vi "input.vi"(8 "error in":errorcluster, 10 "data table in":T1, 11 "Scan Engine runtime in":refnum<class "Scan Engine runtime.lvclass">) -> (0 "error out":errorcluster, 2 "data table out":T1, 3 "Scan Engine runtime out":refnum<class "Scan Engine runtime.lvclass">)   [LabVIEW 2014, in "Scan Engine runtime.lvclass"]
doc: "Provides an interface for reading data from a module at runtime. While this interface performs no operations, a child should provide an override which may read from any open sessions, references, or interfaces."
uses:
  Scan Engine runtime.lvclass
  <vilib>/NI/Tag Bus/table/data table.lvlib
  <vilib>/NI/Tag Bus/table/data polymorphs/write one/write Boolean.vi
  <vilib>/NI/Tag Bus/table/data polymorphs/write one/write U8.vi
  <vilib>/NI/Tag Bus/table/data polymorphs/write one/write U16.vi
  <vilib>/NI/Tag Bus/table/data polymorphs/write one/write U32.vi
  <vilib>/NI/Tag Bus/table/data polymorphs/write one/write I8.vi
  <vilib>/NI/Tag Bus/table/data polymorphs/write one/write I16.vi
  <vilib>/NI/Tag Bus/table/data polymorphs/write one/write I32.vi
  <vilib>/NI/Tag Bus/table/data polymorphs/write one/write I64.vi
  <vilib>/NI/Tag Bus/table/data polymorphs/write one/write Single.vi
  <vilib>/NI/Tag Bus/table/data polymorphs/write one/write Double.vi
  <vilib>/NI/Tag Bus/table/data polymorphs/write one/write U64.vi
  <vilib>/NI/Tag Bus/table/data polymorphs/write many/write Doubles.vi
  <vilib>/NI/Tag Bus/table/data polymorphs/write many/write Singles.vi
  <vilib>/NI/Tag Bus/table/data polymorphs/write many/write I64s.vi
  <vilib>/NI/Tag Bus/table/data polymorphs/write many/write I32s.vi
  <vilib>/NI/Tag Bus/table/data polymorphs/write many/write I16s.vi
  <vilib>/NI/Tag Bus/table/data polymorphs/write many/write I8s.vi
  <vilib>/NI/Tag Bus/table/data polymorphs/write many/write U64s.vi
  <vilib>/NI/Tag Bus/table/data polymorphs/write many/write U32s.vi
  <vilib>/NI/Tag Bus/table/data polymorphs/write many/write U16s.vi
  <vilib>/NI/Tag Bus/table/data polymorphs/write many/write U8s.vi
  <vilib>/NI/Tag Bus/table/data polymorphs/write many/write Booleans.vi
  <vilib>/NI/Tag Bus/table/data table.ctl
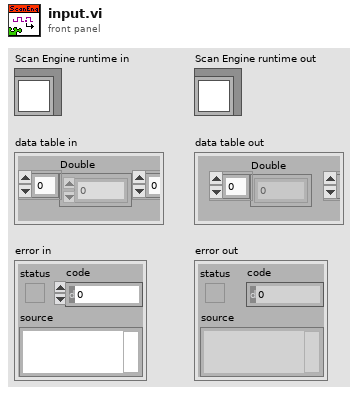
[diagram p1: front panel]
types:
  T1 = typedef "tag bus.lvlib/data table.lvlib/data table.ctl" = cluster{"Double":dbl[], "Single":sgl[], "I64":i64[], "I32":i32[], "I16":i16[], "I8":i8[], "U64":u64[], "U32":u32[], "U16":u16[], "U8":u8[], "Boolean":bool[], "String":string[], "Array of Double":cluster{"DBL Array":dbl[]}[], "Array of Single":cluster{"SGL Array":sgl[]}[], "Array of I64":cluster{"I64 Array":i64[]}[], "Array of I32":cluster{"I32 Array":i32[]}[], "Array of I16":cluster{"I16 Array":i16[]}[], "Array of I8":cluster{"I8 Array":i8[]}[], "Array of U64":cluster{"U64 Array":u64[]}[], "Array of U32":cluster{"U32 Array":u32[]}[], "Array of U16":cluster{"U16 Array":u16[]}[], "Array of U8":cluster{"U8 Array":u8[]}[], "Array of Boolean":cluster{"Boolean Array":bool[]}[], "Array of String":cluster{"String Array":string[]}[]}
  T2 = typedef "IO_index_map.ctl" = cluster{"module_ref":refnum<k21>, "data type":T3, "IO_variable_info":T4[], "IO_module_index_array":i32[], "IO_table_index":i32[], "IO_table_index_ordered":i32[], "use_scanned_methods":bool}
  T3 = typedef "tag bus.lvlib/tag descriptor.lvclass/Data Type.ctl" = enum16{"Double", "Single", "I64", "I32", "I16", "I8", "U64", "U32", "U16", "U8", "Boolean", "String", "Array of Double", "Array of Single", "Array of I64", "Array of I32", "Array of I16", "Array of I8", "Array of U64", "Array of U32", "Array of U16", "Array of U8", "Array of Boolean", "Array of String"}
  T4 = typedef "Scan Engine runtime.lvclass/Index Map.ctl" = cluster{"data type":T3, "variable ref":refnum<k21>, "index":i32, "IO Var":bool, "module_index":i32}
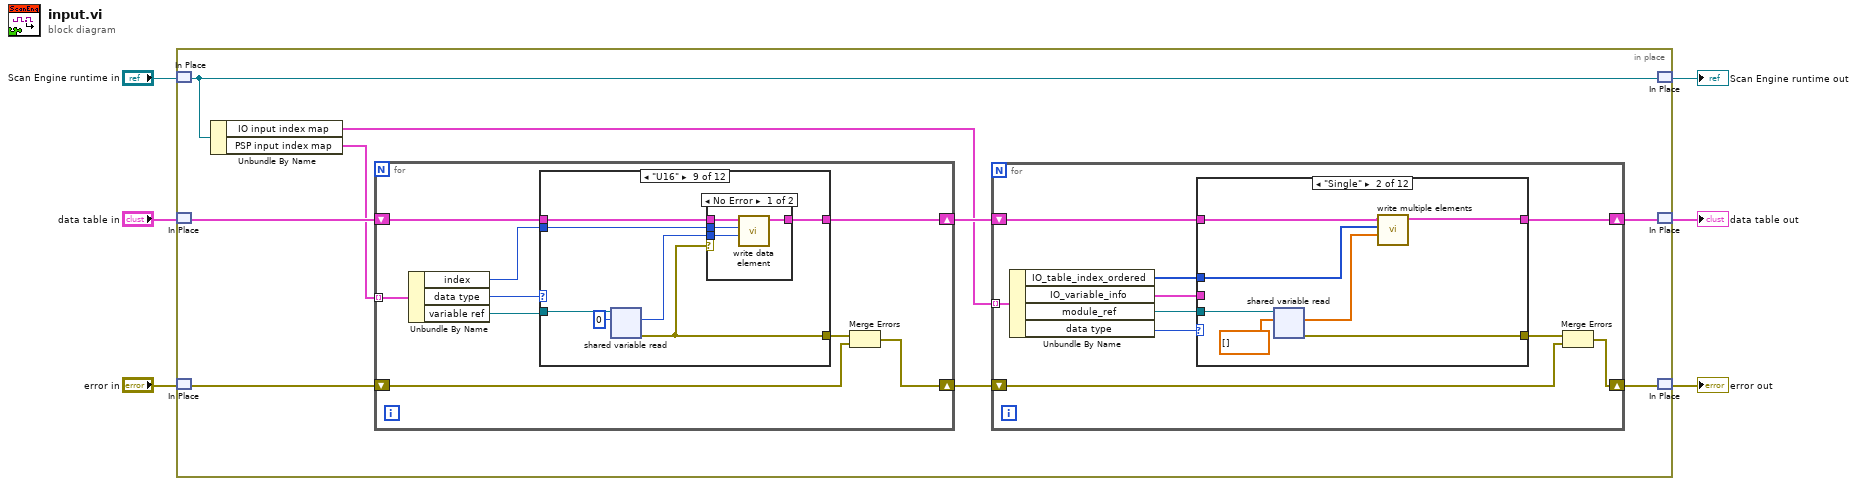
[diagram p0: block diagram]
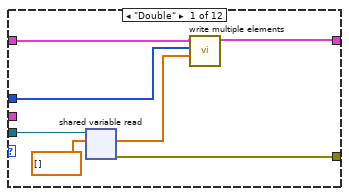
[diagram p2: hidden frame]
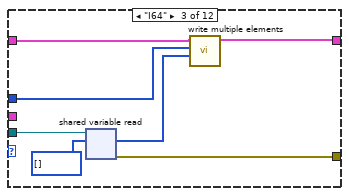
[diagram p3: hidden frame]
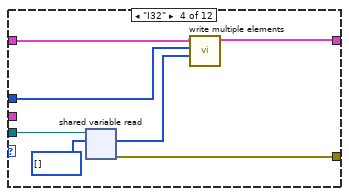
[diagram p4: hidden frame]
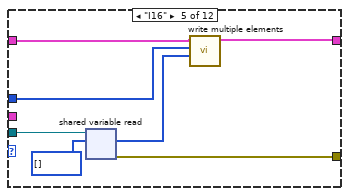
[diagram p5: hidden frame]
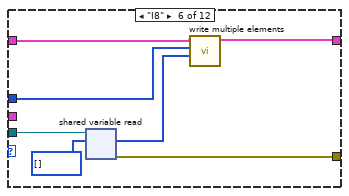
[diagram p6: hidden frame]
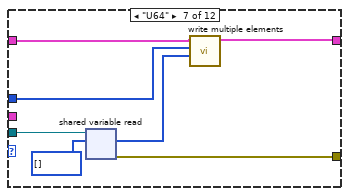
[diagram p7: hidden frame]
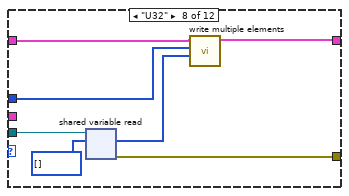
[diagram p8: hidden frame]
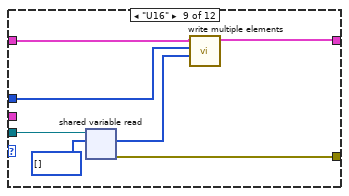
[diagram p9: hidden frame]
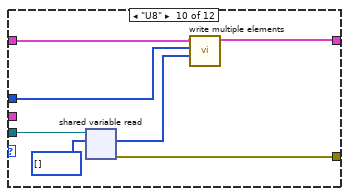
[diagram p10: hidden frame]
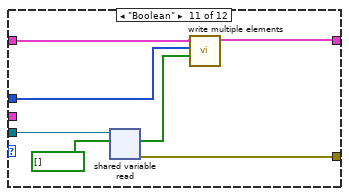
[diagram p11: hidden frame]
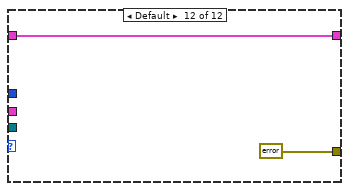
[diagram p12: hidden frame]
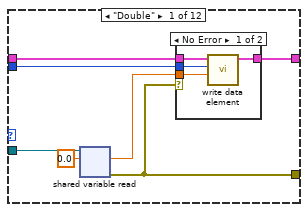
[diagram p13: hidden frame]
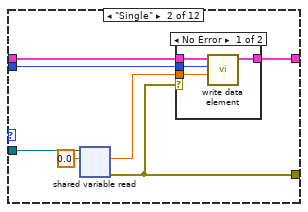
[diagram p15: hidden frame]
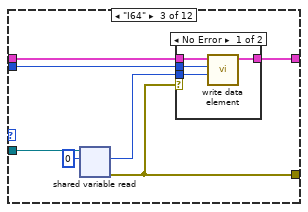
[diagram p17: hidden frame]
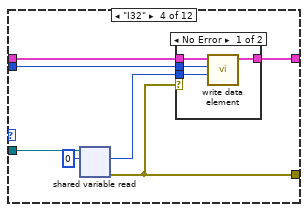
[diagram p19: hidden frame]
diagram:
  n1 = in-place {
    n2 = in-place-match #1("Scan Engine runtime in") -> (w15:refnum<class "Scan Engine runtime.lvclass">)
    n3 = in-place-match #2("data table in") -> (w14:T1)
    n4 = in-place-match #3("error in") -> (w13:errorcluster)
    n5 = Unbundle By Name(w15) -> ("IO input index map"=w10:T2[], "PSP input index map"=w9:T4[])
    n6 = for {
      shift-right: [w110] -> w12
      shift-left: w14 -> [w111]
      shift-right: [w105] -> w8
      shift-left: w13 -> [w106]
      tunnel: w9 -> [w113] mode=indexing
      n7 = Unbundle By Name(w113) -> ("index"=w109:i32, "data type"=w112:T3, "variable ref"=w108:refnum<k21>)
      n8 = case shown="\"U16\"" w112 {
        tunnel: w111 -> [w120 w132 w144 w156 w168 w180 w192 w204 w216 w228 w240 w247]
        tunnel: [w119 w131 w143 w155 w167 w179 w191 w203 w215 w227 w239 w247] -> w110
        tunnel: w109 -> [w118 w130 w142 w154 w166 w178 w190 w202 w214 w226 w238 _]
        tunnel: w108 -> [w117 w129 w141 w153 w165 w177 w189 w201 w213 w225 w237 _]
        tunnel: [w114 w126 w138 w150 w162 w174 w186 w198 w210 w222 w234 errorcluster {"status"=FALSE, "code"=0, "source"=""} ("error IO")] -> w107
        frame "Double" {
          n9 = shared-variable-read(w117, 0.0) -> (w114:errorcluster, w115:dbl)  [unwired: 1 in, 1 out]
          n10 = case shown="No Error" w114 {
            tunnel: w120 -> [w124 w125]
            tunnel: [w123 w125] -> w119
            tunnel: w118 -> [w122 _]
            tunnel: w115 -> [w121 _]
            frame No Error {
              n11 = call-poly <vilib>:"write data element.vi"("value"=w121, "index"=w122, "data table in"=w124) -> ("data table out"=w123:T1)  [unwired: 8 in]
            }
            frame Error {
            }
          }
        }
        frame "Single" {
          n12 = shared-variable-read(w129, sgl 0.0) -> (w126:errorcluster, w127:sgl)  [unwired: 1 in, 1 out]
          n13 = case shown="No Error" w126 {
            tunnel: w132 -> [w136 w137]
            tunnel: [w135 w137] -> w131
            tunnel: w130 -> [w134 _]
            tunnel: w127 -> [w133 _]
            frame No Error {
              n14 = call-poly <vilib>:"write data element.vi"("value"=w133, "index"=w134, "data table in"=w136) -> ("data table out"=w135:T1)  [unwired: 8 in]
            }
            frame Error {
            }
          }
        }
        frame "I64" {
          n15 = shared-variable-read(w141, i64 0) -> (w138:errorcluster, w139:i64)  [unwired: 1 in, 1 out]
          n16 = case shown="No Error" w138 {
            tunnel: w144 -> [w148 w149]
            tunnel: [w147 w149] -> w143
            tunnel: w142 -> [w146 _]
            tunnel: w139 -> [w145 _]
            frame No Error {
              n17 = call-poly <vilib>:"write data element.vi"("value"=w145, "index"=w146, "data table in"=w148) -> ("data table out"=w147:T1)  [unwired: 8 in]
            }
            frame Error {
            }
          }
        }
        frame "I32" {
          n18 = shared-variable-read(w153, 0) -> (w150:errorcluster, w151:i32)  [unwired: 1 in, 1 out]
          n19 = case shown="No Error" w150 {
            tunnel: w156 -> [w160 w161]
            tunnel: [w159 w161] -> w155
            tunnel: w154 -> [w158 _]
            tunnel: w151 -> [w157 _]
            frame No Error {
              n20 = call-poly <vilib>:"write data element.vi"("value"=w157, "index"=w158, "data table in"=w160) -> ("data table out"=w159:T1)  [unwired: 8 in]
            }
            frame Error {
            }
          }
        }
        frame "I16" {
          n21 = shared-variable-read(w165, i16 0) -> (w162:errorcluster, w163:i16)  [unwired: 1 in, 1 out]
          n22 = case shown="No Error" w162 {
            tunnel: w168 -> [w172 w173]
            tunnel: [w171 w173] -> w167
            tunnel: w166 -> [w170 _]
            tunnel: w163 -> [w169 _]
            frame No Error {
              n23 = call-poly <vilib>:"write data element.vi"("value"=w169, "index"=w170, "data table in"=w172) -> ("data table out"=w171:T1)  [unwired: 8 in]
            }
            frame Error {
            }
          }
        }
        frame "I8" {
          n24 = shared-variable-read(w177, i8 0) -> (w174:errorcluster, w175:i8)  [unwired: 1 in, 1 out]
          n25 = case shown="No Error" w174 {
            tunnel: w180 -> [w184 w185]
            tunnel: [w183 w185] -> w179
            tunnel: w178 -> [w182 _]
            tunnel: w175 -> [w181 _]
            frame No Error {
              n26 = call-poly <vilib>:"write data element.vi"("value"=w181, "index"=w182, "data table in"=w184) -> ("data table out"=w183:T1)  [unwired: 8 in]
            }
            frame Error {
            }
          }
        }
        frame "U64" {
          n27 = shared-variable-read(w189, u64 0) -> (w186:errorcluster, w187:u64)  [unwired: 1 in, 1 out]
          n28 = case shown="No Error" w186 {
            tunnel: w192 -> [w196 w197]
            tunnel: [w195 w197] -> w191
            tunnel: w190 -> [w194 _]
            tunnel: w187 -> [w193 _]
            frame No Error {
              n29 = call-poly <vilib>:"write data element.vi"("value"=w193, "index"=w194, "data table in"=w196) -> ("data table out"=w195:T1)  [unwired: 8 in]
            }
            frame Error {
            }
          }
        }
        frame "U32" {
          n30 = shared-variable-read(w201, u32 0) -> (w198:errorcluster, w199:u32)  [unwired: 1 in, 1 out]
          n31 = case shown="No Error" w198 {
            tunnel: w204 -> [w208 w209]
            tunnel: [w207 w209] -> w203
            tunnel: w202 -> [w206 _]
            tunnel: w199 -> [w205 _]
            frame No Error {
              n32 = call-poly <vilib>:"write data element.vi"("value"=w205, "index"=w206, "data table in"=w208) -> ("data table out"=w207:T1)  [unwired: 8 in]
            }
            frame Error {
            }
          }
        }
        frame "U16" {
          n33 = shared-variable-read(w213, u16 0) -> (w210:errorcluster, w211:u16)  [unwired: 1 in, 1 out]
          n34 = case shown="No Error" w210 {
            tunnel: w216 -> [w220 w221]
            tunnel: [w219 w221] -> w215
            tunnel: w214 -> [w218 _]
            tunnel: w211 -> [w217 _]
            frame No Error {
              n35 = call-poly <vilib>:"write data element.vi"("value"=w217, "index"=w218, "data table in"=w220) -> ("data table out"=w219:T1)  [unwired: 8 in]
            }
            frame Error {
            }
          }
        }
        frame "U8" {
          n36 = shared-variable-read(w225, u8 0) -> (w222:errorcluster, w223:u8)  [unwired: 1 in, 1 out]
          n37 = case shown="No Error" w222 {
            tunnel: w228 -> [w232 w233]
            tunnel: [w231 w233] -> w227
            tunnel: w226 -> [w230 _]
            tunnel: w223 -> [w229 _]
            frame No Error {
              n38 = call-poly <vilib>:"write data element.vi"("value"=w229, "index"=w230, "data table in"=w232) -> ("data table out"=w231:T1)  [unwired: 8 in]
            }
            frame Error {
            }
          }
        }
        frame "Boolean" {
          n39 = shared-variable-read(w237, FALSE) -> (w234:errorcluster, w235:bool)  [unwired: 1 in, 1 out]
          n40 = case shown="No Error" w234 {
            tunnel: w240 -> [w244 w245]
            tunnel: [w243 w245] -> w239
            tunnel: w238 -> [w242 _]
            tunnel: w235 -> [w241 _]
            frame No Error {
              n41 = call-poly <vilib>:"write data element.vi"("value"=w241, "index"=w242, "data table in"=w244) -> ("data table out"=w243:T1)  [unwired: 8 in]
            }
            frame Error {
            }
          }
        }
        frame Default {
        }
      }
      n42 = Merge Errors(w107, w106) -> (w105:errorcluster)
    }
    n43 = for {
      shift-right: [w23] -> w11
      shift-left: w12 -> [w24]
      shift-right: [w20] -> w7
      shift-left: w8 -> [w21]
      tunnel: w10 -> [w25] mode=indexing
      n44 = Unbundle By Name(w25) -> ("IO_table_index_ordered"=w17:i32[], "IO_variable_info"=w16:T4[], "module_ref"=w19:refnum<k21>, "data type"=w18:T3)
      n45 = case shown="\"Single\"" w18 {
        tunnel: w24 -> [w28 w35 w42 w49 w56 w63 w70 w77 w84 w91 w98 w104]
        tunnel: [w29 w36 w43 w50 w57 w64 w71 w78 w85 w92 w99 w104] -> w23
        tunnel: w19 -> [w32 w39 w46 w53 w60 w67 w74 w81 w88 w95 w102 _]
        tunnel: [w31 w38 w45 w52 w59 w66 w73 w80 w87 w94 w101 errorcluster {"status"=FALSE, "code"=0, "source"=""} ("error IO")] -> w22
        tunnel: w17 -> [w27 w34 w41 w48 w55 w62 w69 w76 w83 w90 w97 _]
        tunnel: w16 -> [_ _ _ _ _ _ _ _ _ _ _ _]
        frame "Double" {
          n46 = shared-variable-read(w32, dbl[] []) -> (w31:errorcluster, w26:dbl[])  [unwired: 1 in, 1 out]
          n47 = call-poly <vilib>:"write multiple elements.vi"("values"=w26, "indices"=w27, "data table in"=w28) -> ("data table out"=w29:T1)  [unwired: 8 in]
        }
        frame "Single" {
          n48 = shared-variable-read(w39, sgl[] []) -> (w38:errorcluster, w33:sgl[])  [unwired: 1 in, 1 out]
          n49 = call-poly <vilib>:"write multiple elements.vi"("values"=w33, "indices"=w34, "data table in"=w35) -> ("data table out"=w36:T1)  [unwired: 8 in]
        }
        frame "I64" {
          n50 = shared-variable-read(w46, i64[] []) -> (w45:errorcluster, w40:i64[])  [unwired: 1 in, 1 out]
          n51 = call-poly <vilib>:"write multiple elements.vi"("values"=w40, "indices"=w41, "data table in"=w42) -> ("data table out"=w43:T1)  [unwired: 8 in]
        }
        frame "I32" {
          n52 = shared-variable-read(w53, i32[] []) -> (w52:errorcluster, w47:i32[])  [unwired: 1 in, 1 out]
          n53 = call-poly <vilib>:"write multiple elements.vi"("values"=w47, "indices"=w48, "data table in"=w49) -> ("data table out"=w50:T1)  [unwired: 8 in]
        }
        frame "I16" {
          n54 = shared-variable-read(w60, i16[] []) -> (w59:errorcluster, w54:i16[])  [unwired: 1 in, 1 out]
          n55 = call-poly <vilib>:"write multiple elements.vi"("values"=w54, "indices"=w55, "data table in"=w56) -> ("data table out"=w57:T1)  [unwired: 8 in]
        }
        frame "I8" {
          n56 = shared-variable-read(w67, i8[] []) -> (w66:errorcluster, w61:i8[])  [unwired: 1 in, 1 out]
          n57 = call-poly <vilib>:"write multiple elements.vi"("values"=w61, "indices"=w62, "data table in"=w63) -> ("data table out"=w64:T1)  [unwired: 8 in]
        }
        frame "U64" {
          n58 = shared-variable-read(w74, u64[] []) -> (w73:errorcluster, w68:u64[])  [unwired: 1 in, 1 out]
          n59 = call-poly <vilib>:"write multiple elements.vi"("values"=w68, "indices"=w69, "data table in"=w70) -> ("data table out"=w71:T1)  [unwired: 8 in]
        }
        frame "U32" {
          n60 = shared-variable-read(w81, u32[] []) -> (w80:errorcluster, w75:u32[])  [unwired: 1 in, 1 out]
          n61 = call-poly <vilib>:"write multiple elements.vi"("values"=w75, "indices"=w76, "data table in"=w77) -> ("data table out"=w78:T1)  [unwired: 8 in]
        }
        frame "U16" {
          n62 = shared-variable-read(w88, u16[] []) -> (w87:errorcluster, w82:u16[])  [unwired: 1 in, 1 out]
          n63 = call-poly <vilib>:"write multiple elements.vi"("values"=w82, "indices"=w83, "data table in"=w84) -> ("data table out"=w85:T1)  [unwired: 8 in]
        }
        frame "U8" {
          n64 = shared-variable-read(w95, u8[] []) -> (w94:errorcluster, w89:u8[])  [unwired: 1 in, 1 out]
          n65 = call-poly <vilib>:"write multiple elements.vi"("values"=w89, "indices"=w90, "data table in"=w91) -> ("data table out"=w92:T1)  [unwired: 8 in]
        }
        frame "Boolean" {
          n66 = shared-variable-read(w102, bool[] []) -> (w101:errorcluster, w96:bool[])  [unwired: 1 in, 1 out]
          n67 = call-poly <vilib>:"write multiple elements.vi"("values"=w96, "indices"=w97, "data table in"=w98) -> ("data table out"=w99:T1)  [unwired: 8 in]
        }
        frame Default {
        }
      }
      n68 = Merge Errors(w22, w21) -> (w20:errorcluster)
    }
    n69 = in-place-match #1(w15) -> (→"Scan Engine runtime out":refnum<class "Scan Engine runtime.lvclass">)
    n70 = in-place-match #2(w11) -> (→"data table out":T1)
    n71 = in-place-match #3(w7) -> (→"error out":errorcluster)
  }
